vi "Ctor.vi"(8 "error in (no error)":errorcluster, 11 "PlatformArrayPanel in":refnum<class "PlatformArrayPanel.lvclass">) -> (0 "error out":errorcluster, 3 "PlatformArrayPanel out":refnum<class "PlatformArrayPanel.lvclass">)   [LabVIEW 2020, in "PicoG-App.lvlib" / "PlatformArrayPanel.lvclass"]
uses:
  PlatformArrayPanel.lvclass
  <vilib>/IlluminatedG/IG OOPanel/OOPanel/ArrayPanel/ArrayPanel.lvclass
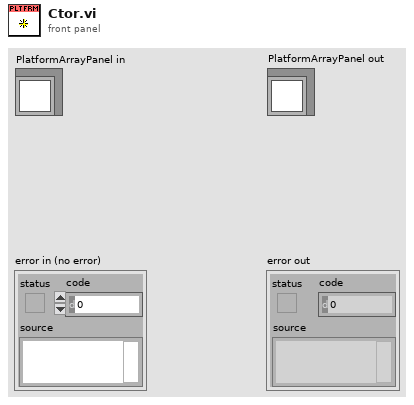
[diagram p1: front panel]
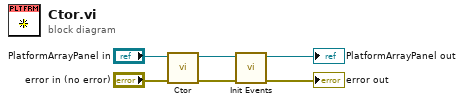
[diagram p0: block diagram]
diagram:
  n1 = call-parent "Ctor.vi"("error in (no error)"="error in (no error)", "ArrayPanel in"="PlatformArrayPanel in") -> ("error out"=w2:errorcluster, "ArrayPanel out"=w1:refnum<class "PlatformArrayPanel.lvclass">)  [unwired: 8 in]
  n2 = call "Init Events.vi"("error in (no error)"=w2, "PlatformArrayPanel in"=w1) -> ("error out"=→"error out":errorcluster, "PlatformArrayPanel out"=→"PlatformArrayPanel out":refnum<class "PlatformArrayPanel.lvclass">)  [unwired: 8 in]
